vi "xiC - IMAQ - CloseWindow.vi"(7 "VI Refnum":refnum<vi>, 11 "error in (no error)":errorcluster) -> (3 "error out":errorcluster)   [LabVIEW 2018]
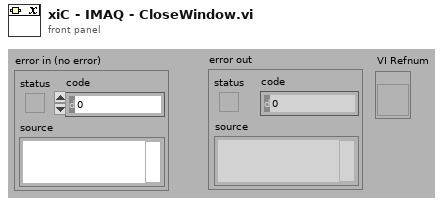
[diagram p1: front panel]
types:
  T1 = enum32{"invalid app kind", "Development System", "Run Time System", "Student Edition", "Embedded LabVIEW", "Evaluation", "Custom"}
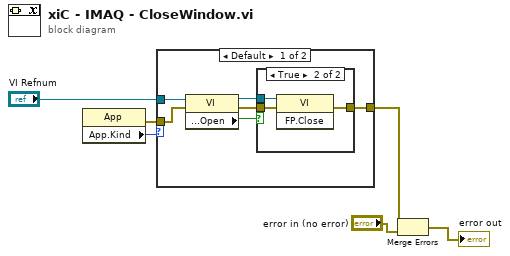
[diagram p0: block diagram]
diagram:
  n1 = property class="App"() -> (error out=w5:errorcluster, "App.Kind"=w6:T1)  [unwired: 2 in, 1 out]
  n2 = case shown="Default" w6 {
    tunnel: "VI Refnum" -> [w9 _]
    tunnel: w5 -> [w8 w17]
    tunnel: [w7 w17] -> w4
    frame Default {
      n3 = property class="VI"(reference=w9, error in=w8) -> (reference out=w11:refnum<vi>, error out=w10:errorcluster, "Front Panel.Open"=w12:bool)
      n4 = case shown="True" w12 {
        tunnel: [w13 w16] -> w7
        tunnel: w10 -> [w13 w15]
        tunnel: w11 -> [_ w14]
        frame False {
        }
        frame True {
          n5 = invoke class="VI" method="FP.Close"(reference=w14, error in=w15) -> (error out=w16:errorcluster)  [unwired: 1 in, 2 out]
        }
      }
    }
    frame "Development System" {
    }
  }
  n6 = Merge Errors(w4, "error in (no error)") -> (→"error out":errorcluster)
